vi "ASK Receiver.vi"() -> ()   [LabVIEW 2015]
uses:
  <vilib>/addons/Modulation/Analog/support/mod_Set Error Source.vi
  <vilib>/addons/Modulation/Digital/General/MT Generate ASK system parameters (M).vi
  <vilib>/addons/Modulation/Digital/Support/Common/Validators/mod_Generate Filter Coefficients Validate.vi
  <vilib>/addons/Modulation/Digital/General/subVIs/mod_Generate Filter Coefficients.vi
  <instrlib>/niUSRP/niUSRP Fetch Rx Data (CDB Cluster).vi
  <vilib>/addons/Modulation/niDMT.lvlib
panel:
  in  "Tab Control 3":enum32{"Page 1", "Page 2"}(tab)
  out "coerced IQ rate":dbl=100000.0 format="%#_6p"
  out "coerced carrier frequency":dbl=100000.0 format="%#_6p"
  out "coerced gain":dbl format="%#_6f"
  in  "Tab Control 2":enum32{"Page 1", "Page 2"}(tab)
  in  "device names":refnum<k15>
  in  "M-ASK (2)":i32=2
  in  "pulse shaping filter (none)":T1(ring)
  in  "IQ rate":dbl=100000.0 format="%#_6p"
  in  "number of samples":i64=1000
  in  "carrier frequency":dbl=100000.0 format="%#_6p"
  in  "gain":dbl format="%#_6f"
  in  "active antenna":string
  in  "Stop":bool
  in  "synchronization parameters":T2 {"sync sequence" format="%.2f"}
  in  "Tab Control":enum32{"Graphs", "Constellation"}(tab)
  out "Waveform Graph":cluster{"t0":dbl, "dt":dbl, "Y":dbl[]}[](graph)
  out "Waveform Graph 2":i8[](graph)
  out "XY Graph":T3(graph)
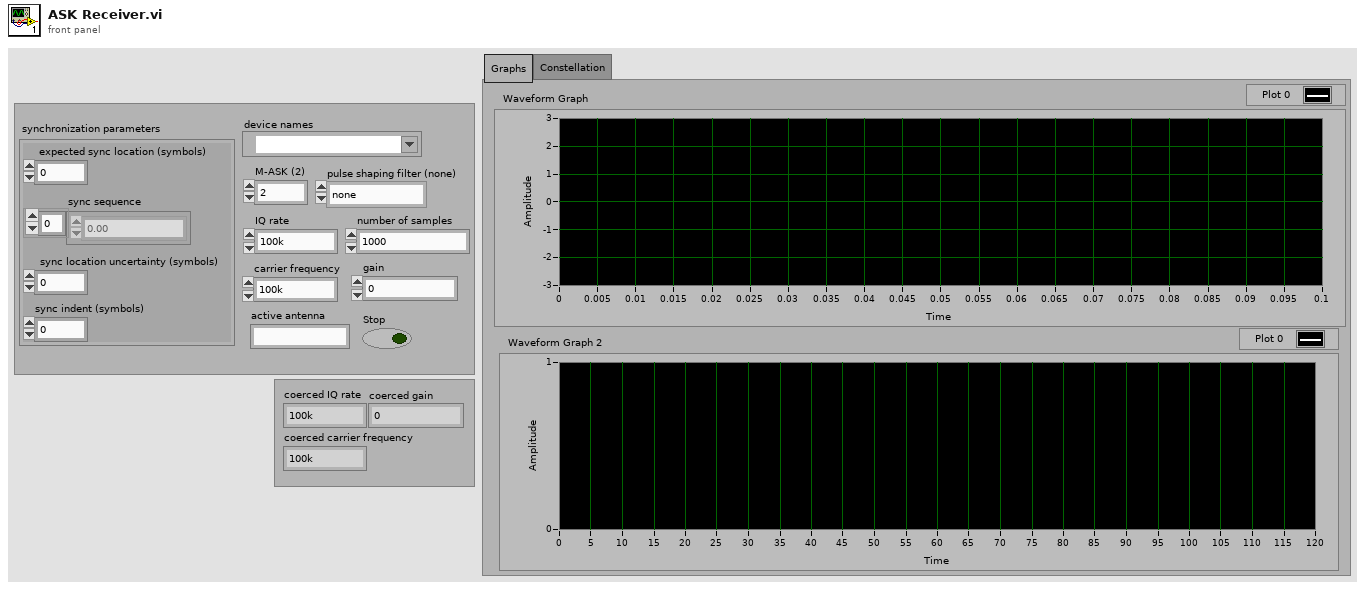
[diagram p1: front panel]
types:
  T1 = enum16{"none", "Raised Cosine", "Root Raised Cos", "Gaussian"}
  T2 = cluster{"expected sync location (symbols)":i32, "sync sequence":cdb[], "sync location uncertainty (symbols)":i32, "sync indent (symbols)":i32}
  T3 = cluster{"constellation":dbl[], "oversampled data":dbl[]}[]
  T4 = enum16{"FSK", "PSK", "QAM", "MSK", "PAM", "ASK", "CPM"}
  T5 = cluster{"samples per symbol (16)":i32, "symbol map":cdb[]}
  T6 = typedef "niAMT.lvlib/Complex Data Waveform.ctl" = cluster{"t0":dbl, "dt":dbl, "Y":cdb[]}
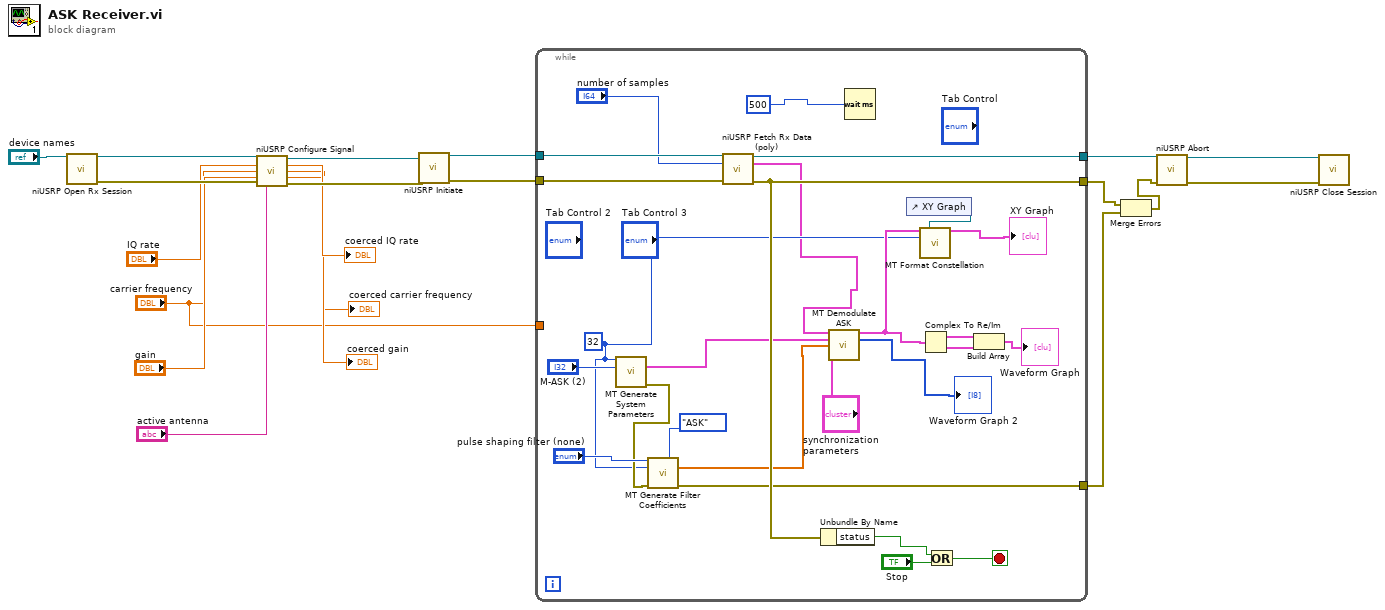
[diagram p0: block diagram]
diagram:
  n1 = call <instrlib>:"niUSRP Open Rx Session.vi"("device names"="device names") -> ("session handle out"=w19:refnum<k15>, "error out"=w17:errorcluster)  [unwired: 13 in]
  n2 = call <instrlib>:"niUSRP Configure Signal.vi"("session handle"=w19, "IQ rate"="IQ rate", "carrier frequency"="carrier frequency", "gain"="gain", "error in (no error)"=w17, "active antenna"="active antenna") -> ("session handle out"=w18:refnum<k15>, "coerced IQ rate"=→"coerced IQ rate":dbl, "coerced carrier frequency"=→"coerced carrier frequency":dbl, "coerced gain"=→"coerced gain":dbl, "error out"=w16:errorcluster)  [unwired: 5 in]
  n3 = call <instrlib>:"niUSRP Initiate.vi"("session handle"=w18, "error in (no error)"=w16) -> ("session handle out"=w15:refnum<k15>, "error out"=w12:errorcluster)  [unwired: 12 in]
  n4 = while {
    tunnel: w15 -> [w46]
    tunnel: [w45] -> w14
    tunnel: w12 -> [w44]
    tunnel: [w40] -> w3
    tunnel: "carrier frequency" -> [_]
    tunnel: [w31] -> w2
    stop <- w43 stop-if-true
    w25 = 32 ("samples per symbol (16)")
    n5 = call-poly <vilib>:"MT Generate System Parameters.vi"("samples per symbol (16)"=w25, "M-ASK (2)"="M-ASK (2)") -> ("ASK system parameters"=w36:T5, "error out"=w32:errorcluster)  [unwired: 11 in, 1 out]
    n6 = call <vilib>:"MT Generate Filter Coefficients.vi"("pulse shaping filter (none)"="pulse shaping filter (none)", "modulation type"=T4."ASK", "pulse shaping samples per symbol (16)"=w25, "error in (no error)"=w32) -> ("matched filter coefficients"=w34:dbl[], "error out"=w31:errorcluster)  [unwired: 9 in, 1 out]
    n7 = call-poly <instrlib>:"niUSRP Fetch Rx Data (poly).vi"("session handle"=w46, "number of samples"="number of samples", "error in (no error)"=w44) -> ("session handle out"=w45:refnum<k15>, "data"=w24:cluster{"t0":dbl, "dt":dbl, "Y":cdb[]}, "error out"=w40:errorcluster)  [unwired: 9 in, 1 out]
    n8 = Unbundle By Name(w40) -> ("status"=w41:bool)
    n9 = call <vilib>:"MT Demodulate ASK.vi"("input complex waveform"=w24, "ASK system parameters"=w36, "matched filter coefficients"=w34, "synchronization parameters"="synchronization parameters") -> ("recovered complex waveform"=w27:T6, "output bit stream"=→"Waveform Graph 2":i8[])  [unwired: 7 in, 3 out]
    n10 = Wait (ms)(milliseconds to wait=u32 500) -> ()  [unwired: 1 out]
    n11 = control-ref of="XY Graph"() -> (w21:refnum<vi>)
    n12 = call <vilib>:"MT Format Constellation.vi"("waveform"=w27, "constellation reference"=w21, "samples per symbol"=w25) -> ("constellation graph"=→"XY Graph":T3)  [unwired: 11 in, 1 out]
    n13 = Complex To Re/Im(x + iy=w27) -> (x=w39:cluster{"t0":dbl, "dt":dbl, "Y":dbl[]}, y=w38:cluster{"t0":dbl, "dt":dbl, "Y":dbl[]})
    n14 = Or(x=w41, y="Stop") -> (x .or. y?=w43:bool)
    n15 = Build Array(w39, w38) -> (→"Waveform Graph":cluster{"t0":dbl, "dt":dbl, "Y":dbl[]}[])
  }
  n16 = Merge Errors(w3, w2) -> (w1:errorcluster)
  n17 = call <instrlib>:"niUSRP Abort.vi"("session handle"=w14, "error in (no error)"=w1) -> ("session handle out"=w13:refnum<k15>, "error out"=w11:errorcluster)  [unwired: 12 in]
  n18 = call <instrlib>:"niUSRP Close Session.vi"("session handle"=w13, "error in (no error)"=w11) -> ()  [unwired: 13 in, 1 out]
